vi "例程27-配置文件的创建.vi"() -> ()   [LabVIEW 2016]
uses:
  <vilib>/Utility/config.llb/Write Key (Boolean).vi
  <vilib>/Utility/config.llb/Write Key (String).vi
  <vilib>/Utility/config.llb/Write Key (Path).vi
  <vilib>/Utility/config.llb/Write Key (Double).vi
  <vilib>/Utility/config.llb/NI_LVConfig.lvlib
panel:
  in  "字符串 2":string
  in  "字符串":string
  in  "路径":path
  in  "数值":dbl
  in  "布尔":bool
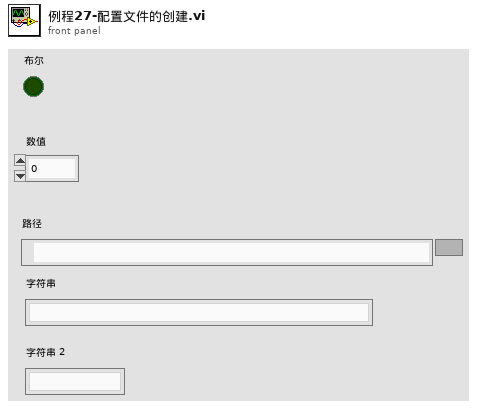
[diagram p1: front panel]
types:
  T1 = typedef "NI_LVConfig.lvlib/Config Data RefNum.ctl" = refnum<k1>
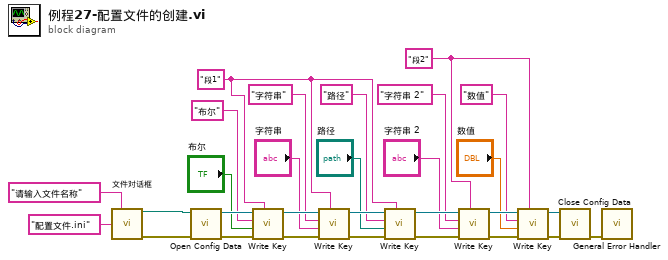
[diagram p0: block diagram]
diagram:
  w5 = "段2" ("section")
  w14 = "段1" ("section")
  n1 = call "文件对话框"("prompt"="请输入文件名称", "default name"="配置文件.ini") -> ("selected path"=w26:path, "error out"=w25:errorcluster)  [unwired: 10 in, 2 out]
  n2 = call <vilib>:"Open Config Data.vi"("error in (no error)"=w25, "configuration file path"=w26) -> ("error out"=w23:errorcluster, "refnum"=w24:T1)  [unwired: 7 in, 1 out]
  n3 = call-poly <vilib>:"Write Key.vi"("section"=w14, "error in (no error)"=w23, "value"="布尔", "key"="布尔", "refnum"=w24) -> ("error out"=w13:errorcluster, "refnum out"=w12:T1)  [unwired: 4 in, 1 out]
  n4 = call-poly <vilib>:"Write Key.vi"("section"=w14, "error in (no error)"=w13, "value"="字符串", "key"="字符串", "refnum"=w12) -> ("error out"=w22:errorcluster, "refnum out"=w21:T1)  [unwired: 4 in, 1 out]
  n5 = call-poly <vilib>:"Write Key.vi"("section"=w14, "error in (no error)"=w22, "value"="路径", "key"="路径", "refnum"=w21) -> ("error out"=w20:errorcluster, "refnum out"=w19:T1)  [unwired: 4 in, 1 out]
  n6 = call-poly <vilib>:"Write Key.vi"("section"=w5, "error in (no error)"=w20, "value"="字符串 2", "key"="字符串 2", "refnum"=w19) -> ("error out"=w18:errorcluster, "refnum out"=w17:T1)  [unwired: 4 in, 1 out]
  n7 = call-poly <vilib>:"Write Key.vi"("section"=w5, "error in (no error)"=w18, "value"="数值", "key"="数值", "refnum"=w17) -> ("error out"=w6:errorcluster, "refnum out"=w4:T1)  [unwired: 4 in, 1 out]
  n8 = call <vilib>:"Close Config Data.vi"("error in (no error)"=w6, "refnum"=w4) -> ("error out"=w29:errorcluster)  [unwired: 8 in, 1 out]
  n9 = call <vilib>:"General Error Handler.vi"("error in (no error)"=w29) -> ()  [unwired: 10 in, 5 out]
